vi "ControlCreate.vi"(0 "__args":T1) -> (1 "__return":cluster{"UID":i32, "Terminal.UID":i32}, 2 "__errStatus":bool, 3 "__errCode":i32, 4 "__errSource":string)   [LabVIEW 2013]
uses:
  <vilib>/Utility/miscctls.llb/LVPointTypeDef.ctl
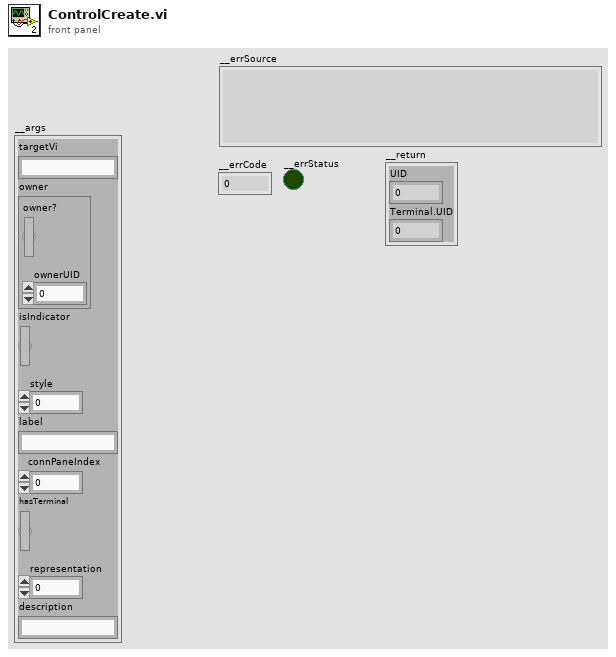
[diagram p1: front panel]
types:
  T1 = cluster{"targetVi":string, "owner":cluster{"owner?":bool, "ownerUID":i32}, "isIndicator":bool, "style":i32, "label":string, "connPaneIndex":i32, "hasTerminal":bool, "representation":i8, "description":string}
  T2 = typedef "LVPointTypeDef.ctl" = cluster{"Horizontal":i16, "Vertical":i16}
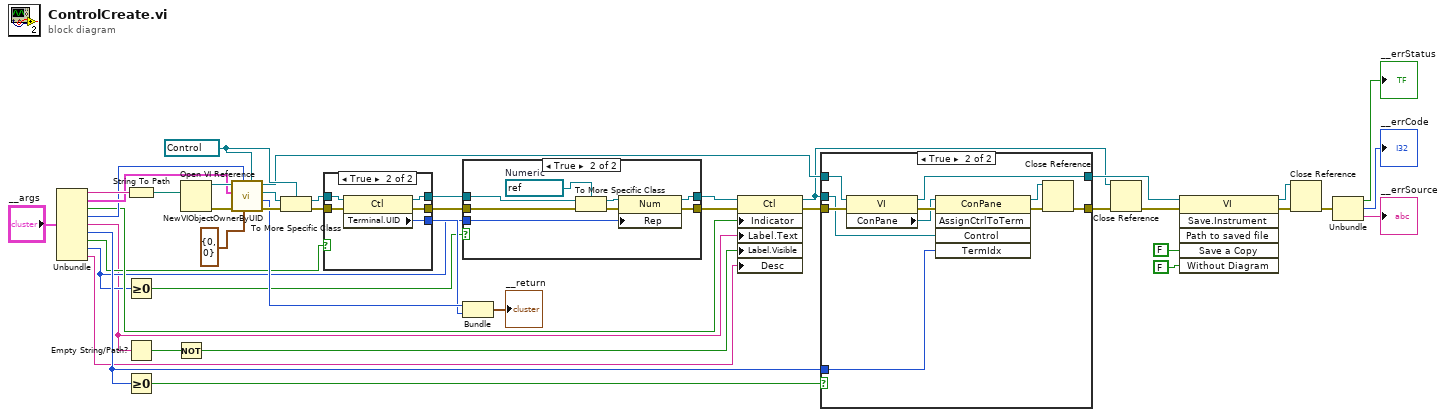
[diagram p0: block diagram]
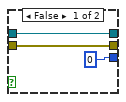
[diagram p3: hidden frame]
diagram:
  w24 = refnum<vi> refnum ("vi object class")
  n1 = Unbundle("__args") -> ("targetVi"=w27:string, "owner"=w26:cluster{"owner?":bool, "ownerUID":i32}, "isIndicator"=w16:bool, "style"=w25:i32, "label"=w4:string, "connPaneIndex"=w18:i32, "hasTerminal"=w14:bool, "representation"=w6:i8, "description"=w3:string)
  n2 = String To Path(string=w27) -> (path=w44:path)
  n3 = Greater Or Equal To 0?(x=w6) -> (x >= 0?=w11:bool)
  n4 = Empty String/Path?(string/path=w4) -> (empty?=w29:bool)
  n5 = Greater Or Equal To 0?(x=w18) -> (x >= 0?=w19:bool)
  n6 = Not(x=w29) -> (.not. x?=w5:bool)
  n7 = Open VI Reference(vi path=w44) -> (vi reference=w34:refnum<vi>, error out=w32:errorcluster)  [unwired: 5 in]
  n8 = call "NewVIObjectOwnerByUID.vi"("vi object class"=w24, "location"=T2 {"Horizontal"=0, "Vertical"=0}, "style"=w25, "error in (no error)"=w32, "owner"=w26, "targetVI"=w34) -> ("error out"=w31:errorcluster, "UID"=w23:i32, "object refnum"=w30:refnum<vi>, "dup targetVI"=w22:refnum<vi>)  [unwired: 2 in]
  n9 = To More Specific Class(target class=w24, reference=w30, error in=w31) -> (specific class reference=w12:refnum<vi>, error out=w13:errorcluster)
  n10 = case shown="True" w14 {
    tunnel: [0 w52] -> w15
    tunnel: [w46 w48] -> w7
    tunnel: [w47 w51] -> w8
    tunnel: w13 -> [w46 w50]
    tunnel: w12 -> [w47 w49]
    frame False {
    }
    frame True {
      n11 = property class="Ctl"(reference=w49, error in=w50) -> (reference out=w51:refnum<vi>, error out=w48:errorcluster, "Terminal.UID"=w52:i32)
    }
  }
  n12 = case shown="True" w11 {
    tunnel: [w54 w62] -> w10
    tunnel: w7 -> [w54 w59]
    tunnel: [w53 w61] -> w9
    tunnel: w8 -> [w53 w60]
    tunnel: w6 -> [_ w55]
    frame False {
    }
    frame True {
      w56 = refnum<vi> refnum  # Numeric
      n13 = To More Specific Class(target class=w56, reference=w60, error in=w59) -> (specific class reference=w57:refnum<vi>, error out=w58:errorcluster)
      n14 = property class="Num"(reference=w57, error in=w58, "Rep"=w55) -> (reference out=w61:refnum<vi>, error out=w62:errorcluster)
    }
  }
  n15 = Bundle("UID"=w23, "Terminal.UID"=w15) -> (→"__return":cluster{"UID":i32, "Terminal.UID":i32})  [unwired: 1 in]
  n16 = property class="Ctl"(reference=w9, error in=w10, "Indicator"=w16, "Label.Text"=w4, "Label.Visible"=w5, "Desc"=w3) -> (reference out=w2:refnum<vi>, error out=w1:errorcluster)
  n17 = case shown="True" w19 {
    tunnel: w22 -> [w64 w74]
    tunnel: w1 -> [w63 w73]
    tunnel: [w64 w72] -> w21
    tunnel: w18 -> [_ w69]
    tunnel: [w63 w67] -> w20
    tunnel: w2 -> [_ w65]
    frame False {
    }
    frame True {
      n18 = property class="VI"(reference=w74, error in=w73) -> (reference out=w72:refnum<vi>, error out=w71:errorcluster, "ConPane"=w70:refnum<vi>)
      n19 = invoke class="ConPane" method="AssignCtrlToTerm"(reference=w70, error in=w71, "Control"=w65, "TermIdx"=w69) -> (reference out=w68:refnum<vi>, error out=w66:errorcluster)  [unwired: 1 in, 3 out]
      n20 = Close Reference(reference=w68, error in (no error)=w66) -> (error out=w67:errorcluster)
    }
  }
  n21 = Close Reference(reference=w2, error in (no error)=w20) -> (error out=w38:errorcluster)
  n22 = invoke class="VI" method="Save.Instrument"(reference=w21, error in=w38, "Save a Copy"=FALSE, "Without Diagram"=FALSE) -> (reference out=w39:refnum<vi>, error out=w37:errorcluster)  [unwired: 2 in, 4 out]
  n23 = Close Reference(reference=w39, error in (no error)=w37) -> (error out=w40:errorcluster)
  n24 = Unbundle(w40) -> ("status"=→"__errStatus":bool, "code"=→"__errCode":i32, "source"=→"__errSource":string)
